vi "Tree Drag Move Row Visualization.vi"(7 "DragStart? (F)":bool, 8 "error in (no error)":errorcluster, 10 "Active Item Tags":string[](array[string]), 11 "TreeRef":refnum<vi>) -> (0 "error out":errorcluster)   [LabVIEW 2020, in "BetterDragAndDrop.lvlib" / "BetterTreeHandle.lvclass"]
uses:
  Classes/BetterTreeHandle/BetterTreeHandle.lvclass
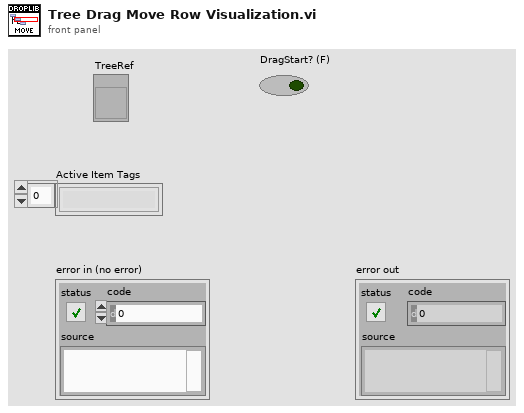
[diagram p1: front panel]
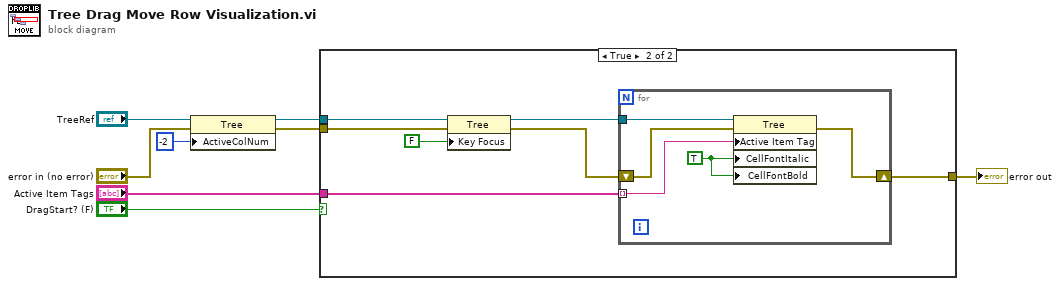
[diagram p0: block diagram]
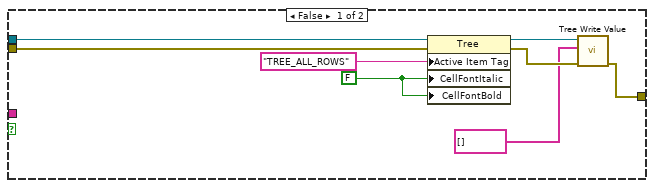
[diagram p2: hidden frame]
diagram:
  n1 = property class="Tree"(reference="TreeRef", error in="error in (no error)", "ActiveColNum"=-2 ("Active Cell:Active Column Number")) -> (reference out=w5:refnum<vi>, error out=w1:errorcluster)
  n2 = case shown="True" "DragStart? (F)" {
    tunnel: w5 -> [w14 w21]
    tunnel: "Active Item Tags" -> [_ w23]
    tunnel: w1 -> [w13 w18]
    tunnel: [w9 w22] -> w7
    frame False {
      w15 = FALSE ("Active Cell:Cell Font:Italic")
      n3 = property class="Tree"(reference=w14, error in=w13, "Active Item Tag"="TREE_ALL_ROWS" ("Active Item:Tag"), "CellFontItalic"=w15, "CellFontBold"=w15) -> (reference out=w12:refnum<vi>, error out=w11:errorcluster)
      n4 = call "Tree Write Value.vi"("error in (no error)"=w11, "Value"=string[] [], "Tree Ref (generic)"=w12) -> ("error out"=w9:errorcluster)  [unwired: 7 in, 1 out]
    }
    frame True {
      n5 = property class="Tree"(reference=w21, error in=w18, "Key Focus"=FALSE) -> (reference out=w19:refnum<vi>, error out=w17:errorcluster)
      n6 = for {
        tunnel: w19 -> [w28]
        tunnel: w23 -> [w27] mode=indexing
        shift-right: [w24] -> w22
        shift-left: w17 -> [w25]
        w26 = TRUE ("Active Cell:Cell Font:Italic")
        n7 = property class="Tree"(reference=w28, error in=w25, "Active Item Tag"=w27, "CellFontItalic"=w26, "CellFontBold"=w26) -> (error out=w24:errorcluster)  [unwired: 1 out]
      }
    }
  }
  "error out" <- w7
